vi "LVRT Serial Init Used.vi"(5 "FPGA Interface":T1, 6 "stop bits (10: 1 bit)":u16(ring)=10 items=["1 bit"=10, "1.5 bits"=15, "2 bits"=20], 7 "Invert Polarity?":bool, 8 "error in (no error)":errorcluster, 9 "parity (0:none)":u16(ring) items=["None", "Odd", "Even", "Mark", "Space"], 10 "data bits (8)":u16=8 min=5 max=8 step=1, 11 "baud rate (9600)":u32=9600) -> (0 "error out":errorcluster, 3 "FPGA Interface 2":T1)   [LabVIEW 2015]
uses:
  fpga-type-def.ctl
  <vilib>/Utility/error.llb/Error Cluster From Error Code.vi
  <vilib>/rvi/errors/niLvFpgaAdjustHostInterfaceError.vi
  <vilib>/rvi/interface/nirviReadWriteControl/nirviReadWriteControl.xnode
  FPGA Bitfiles/Raptorv2_FPGATarget_FPGAMain_QFI8efjbaF8.lvbitx
  FPGA/Main FPGA.vi
  NiFpgaLv.dll
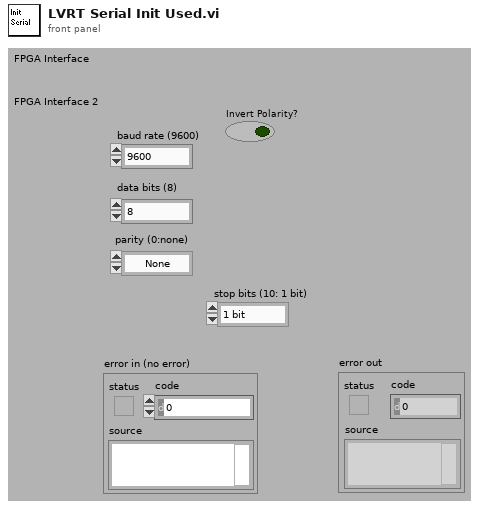
[diagram p1: front panel]
types:
  T1 = typedef "fpga-type-def.ctl" = refnum<k20>
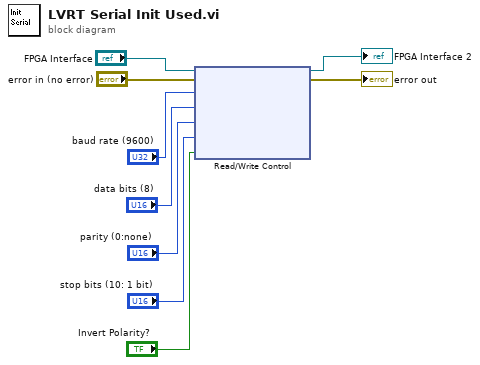
[diagram p0: block diagram]
diagram:
  n1 = xnode "Read/Write Control"("FPGA VI Reference In"="FPGA Interface", "error in"="error in (no error)", "baud rate (9600)"="baud rate (9600)", "data bits (8)"="data bits (8)", "parity (0:none)"="parity (0:none)", "stop bits (10: 1 bit)"="stop bits (10: 1 bit)", "Invert Polarity?"="Invert Polarity?") -> ("FPGA VI Reference Out"=→"FPGA Interface 2":T1, "error out"=→"error out":errorcluster)
